vi "GEA2_RQST_STATUS_QUERY.vi"(0 "ComPort":refnum<visa-resource-name>="COM1", 11 "Error In":errorcluster) -> (3 "Current Status Array":string[][](array[string]), 4 "ACK":bool, 6 "Mode":T1=enum."HighDemand", 8 "Current SetPoint":u8, 10 "CRC Match":bool, 15 "Error Out":errorcluster)   [LabVIEW 2009]
uses:
  HEWH_Mode.ctl
  HEWH Command Type.ctl
panel:
  out "DataReturned":u8[](array[numeric]) format="%.0x"
  # "1=hybrid\n2=stdelect\n3=eheat"
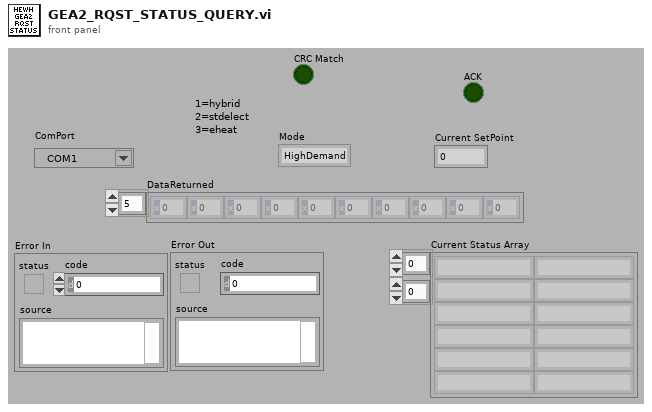
[diagram p1: front panel]
types:
  T1 = typedef "HEWH_Mode.ctl" = enum16{"Hybrid", "StdElectric", "eHeat", "HighDemand", "Vacation"}
  T2 = typedef "HEWH Command Type.ctl" = u8
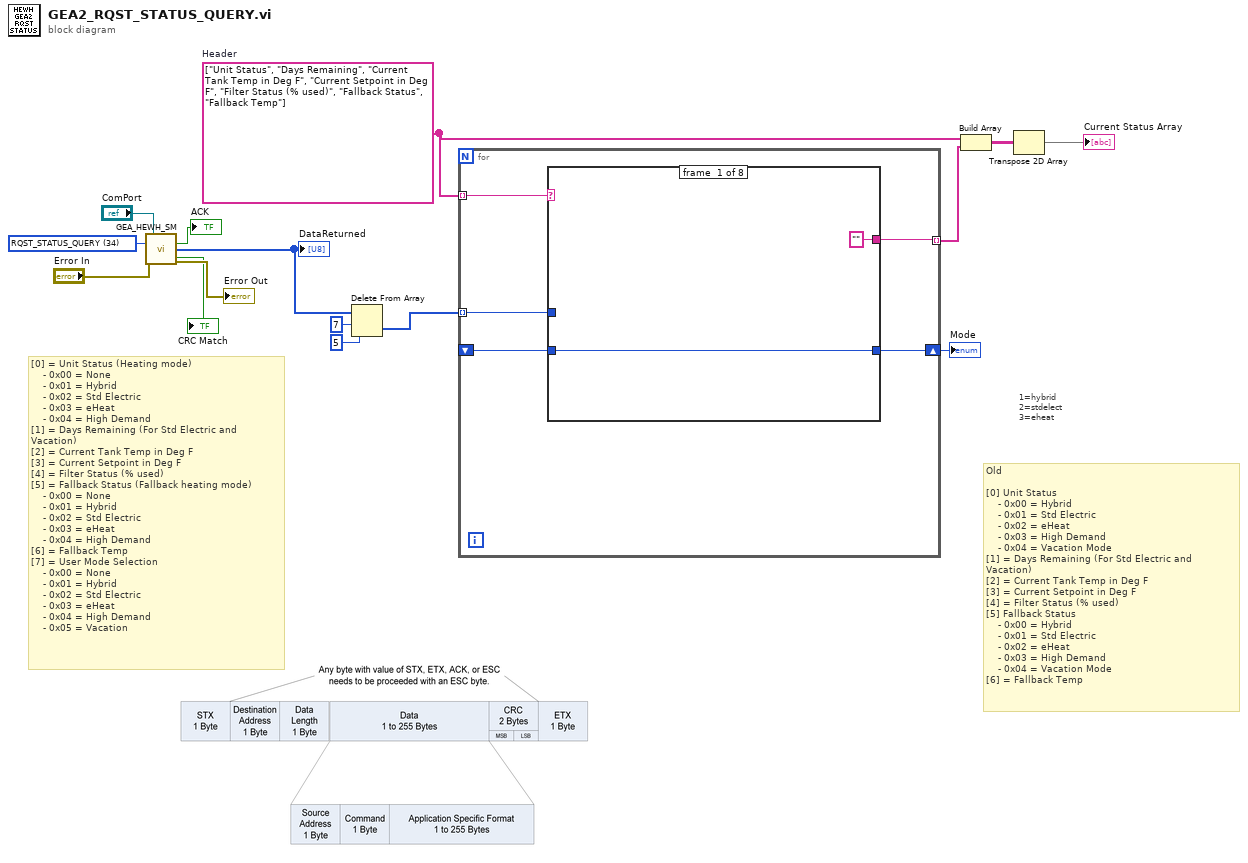
[diagram p0: block diagram]
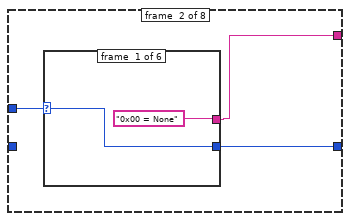
[diagram p2: hidden frame]
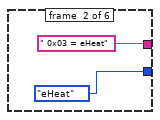
[diagram p3: hidden frame]
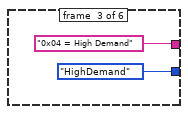
[diagram p4: hidden frame]
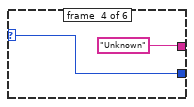
[diagram p5: hidden frame]
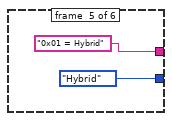
[diagram p6: hidden frame]
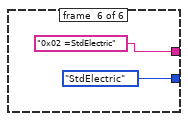
[diagram p7: hidden frame]
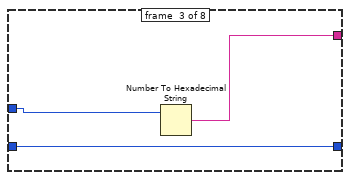
[diagram p8: hidden frame]
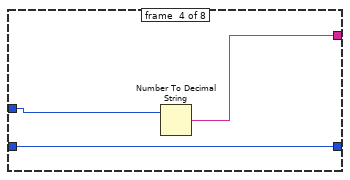
[diagram p9: hidden frame]
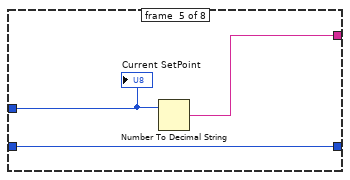
[diagram p10: hidden frame]
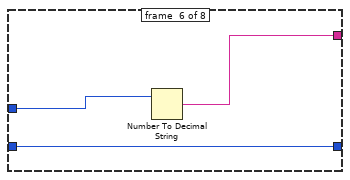
[diagram p11: hidden frame]
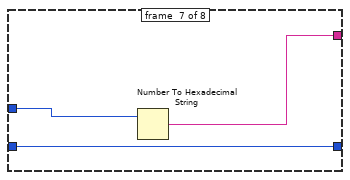
[diagram p12: hidden frame]
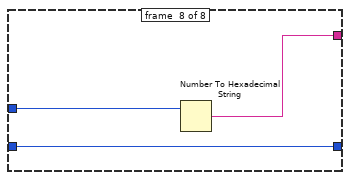
[diagram p13: hidden frame]
diagram:
  w2 = T2 34 items=["RQST_SOFTWARE_VERSION", "RQST_T2_RESISTANCE", "RQST_T3A_RESISTANCE", "RQST_T3B_RESISTANCE", "RQST_T4_RESISTANCE", "RQST_T5_RESISTANCE", "RQST_IDLB_RESISTANCE", "RQST_MODE_SELECT_RESISTANCE", "RQST_DATA_FROM_MEMORY", "RQST_DATA_FROM_DATA_FLASH", "RQST_SS_FAULT_COUNTS", "RQST_OTHER_FAULT_COUNTS", "CMD_CLEAR_FAULT_COUNTS", "RQST_HYPERTERM_OUTPUT_DATA", "CMD_RESET_FILTER_TIMES", "CMD_WRITE_SETPOINTS", "CMD_TURN_ON_OFF_DLB", "CMD_ENTER_EXIT_FCT_MODE", "CMD_SET_LEDS", "CMD_SET_EEV_DRIVE_LINES", "REQ_READ_KEY_STATUS", "RQST_READ_PERSONALITY", "CMD_ENTER_FACT_MODE", "CMD_RESET", "CMD_RESTORE_EEPROM_DEFAULTS", "CMD_SET_MODEL_NUMBER", "CMD_SET_SERIAL_NUMBER", "RQST_MODEL_NUMBER", "RQST_SERIAL_NUMBER", "CMD_TOGGLE_SERVICE_MODE", "CMD_TOGGLE_UE_SERV", "CMD_TOGGLE_LE_SERV", "CMD_REFRESH_SERVICE_TIMEOUTS", "RQST_DSM_OVERRIDE_STATUS", "RQST_STATUS_QUERY", "RQST_HEM_KWH_DATA", "RQST_SERVICE_ERROR_CODES", "RQST_OVERRIDE_STATUS", "CMD_UPDATE_DSM_LEVEL", "CMD_OVERRIDE_STATUS_CHANGED", "CMD_CLEAR_OVERRIDE_STATUS", "CMD_CLEAR_ENERGY_USAGE_CTRS", "CMD_DSM_OVERRIDES", "CMD_UPDATE_MODE", "CMD_SET_PID_P_DENOMINATOR", "CMD_SET_PID_I_DENOM_UNDER_THR", "CMD_SET_PID_I_DENOM_OVER_THR", "CMD_SET_START_POS_UNDER_THR", "CMD_SET_START_POS_OVER_THR", "CMD_SET_EEV_STOP_POSITION", "CMD_SET_AMBIENT_THRESH_1", "CMD_SET_AMBIENT_THRESH_2", "CMD_SET_AMBIENT_THRESH_3", "CMD_SET_PID_LOW_SH_TARGET", "CMD_SET_PID_MID_SH_TARGET", "RQST_PID_PARAMETERS", "CMD_COMP_OFF", "CMD_TOGGLE_FAN", "CMD_RQST_LED_STATUS", "CMD_UE_2_SECONDS", "CMD_LE_2_SECONDS", "CMD_COMP_ON", "CMD_HP_RUN_6MIN", "RQST_TEMP_RANGE", "RQST_VACATION_RANGE", "RQST_STD_ELEC_RANGE", "RQST_WATER_CAPACITY", "CMD_CANCEL_EEV_POSITION", "CMD_EEV_POSITION", "CMD_SET_CURRENTS", "RQST_SUPPORTED_MODES"] ("Command")
  w5 = string[] ["Unit Status", "Days Remaining", "Current Tank Temp in Deg F", "Current Setpoint in Deg F", "Filter Status (% used)", "Fallback Status", "Fallback Temp"]  # Header
  # "[0] = Unit Status (Heating mode)\n    - 0x00 = None\n    - 0x01 = Hybrid\n    - 0x02 = Std Electric\n    - 0x03 = eHeat\n    - 0x04 = High Demand\n[1] = Days Remaining (For Std Electric and Vacation)\n[2] = Current Tank Temp in Deg F\n[3] = Current Setpoint in Deg F\n[4] = Filter Status (% used)\n[5] = Fallback Status (Fallback heating mode)\n    - 0x00 = None\n    - 0x01 = Hybrid\n    - 0x02 = Std Electric\n    - 0x03 = eHeat\n    - 0x04 = High Demand\n[6] = Fallback Temp\n[7] = User Mode Selection\n    - 0x00 = None\n    - 0x01 = Hybrid\n    - 0x02 = Std Electric\n    - 0x03 = eHeat\n    - 0x04 = High Demand\n    - 0x05 = Vacation"
  # "1=hybrid\n2=stdelect\n3=eheat"
  # "Old\n\n[0] Unit Status\n    - 0x00 = Hybrid\n    - 0x01 = Std Electric\n    - 0x02 = eHeat\n    - 0x03 = High Demand\n    - 0x04 = Vacation Mode\n[1] = Days Remaining (For Std Electric and Vacation)\n[2] = Current Tank Temp in Deg F\n[3] = Current Setpoint in Deg F\n[4] = Filter Status (% used)\n[5] Fallback Status\n    - 0x00 = Hybrid\n    - 0x01 = Std Electric\n    - 0x02 = eHeat\n    - 0x03 = High Demand\n    - 0x04 = Vacation Mode\n[6] = Fallback Temp"
  n1 = call "GEA_HEWH_SM.vi"("ComPort"="ComPort", "Command"=w2, "Error In"="Error In") -> ("Read_ACK"=→"ACK":bool, "DataReturned"=w11:u8[], "CRC Match"=→"CRC Match":bool, "Error Out"=→"Error Out":errorcluster)  [unwired: 8 in, 1 out]
  "DataReturned" <- w11
  n2 = Delete From Array(array=w11, length=7, index=5) -> (deleted portion=w1:u8[])  [unwired: 1 out]
  n3 = for {
    tunnel: w5 -> [w20] mode=indexing
    tunnel: w1 -> [w19] mode=indexing
    tunnel: [w18] -> w6 mode=indexing
    shift-right: [w17] -> w7
    shift-left: _ -> [w16]
    n4 = case shown="\"Unit Status\"" w20 {
      tunnel: w19 -> [_ w25 w39 w42 w45 w48 w51 w54]
      tunnel: ["" w24 w40 w43 w46 w49 w52 w55] -> w18
      tunnel: [w21 w23 w38 w41 w44 w47 w50 w53] -> w17
      tunnel: w16 -> [w21 _ w38 w41 w44 w47 w50 w53]
      frame #0 {
      }
      frame #1 {
        n5 = case shown="5, Default" w25 {
          selector: w25 -> [w26 _ _ w32 _ _]
          tunnel: ["0x00 = None" " 0x03 = eHeat" "0x04 = High Demand" "Unknown" "0x01 = Hybrid" "0x02 =StdElectric"] -> w24
          tunnel: [w26 HEWH_Mode."eHeat" ("Mode") HEWH_Mode."HighDemand" ("Mode 2") w32 HEWH_Mode."Hybrid" ("Mode") HEWH_Mode."StdElectric" ("Mode")] -> w23
          frame #0 {
          }
          frame #1 {
          }
          frame #2 {
          }
          frame #3 {
          }
          frame #4 {
          }
          frame #5 {
          }
        }
      }
      frame #2 {
        n6 = Number To Hexadecimal String(2:w39) -> (0:w40:string)  [unwired: 1 in]
      }
      frame #3 {
        n7 = Number To Decimal String(number=w42) -> (decimal integer string=w43:string)  [unwired: 1 in]
      }
      frame #4 {
        n8 = Number To Decimal String(number=w45) -> (decimal integer string=w46:string)  [unwired: 1 in]
        "Current SetPoint" <- w45
      }
      frame #5 {
        n9 = Number To Decimal String(number=w48) -> (decimal integer string=w49:string)  [unwired: 1 in]
      }
      frame #6 {
        n10 = Number To Hexadecimal String(2:w51) -> (0:w52:string)  [unwired: 1 in]
      }
      frame #7 {
        n11 = Number To Hexadecimal String(2:w54) -> (0:w55:string)  [unwired: 1 in]
      }
    }
  }
  "Mode" <- w7
  n12 = Build Array(w5, w6) -> (w4:string[][])
  n13 = Transpose 2D Array(2D array=w4) -> (transposed array=→"Current Status Array":string[][])
